vi "Send Subscription List To Robot.vi"(8 "error in (no error)":errorcluster, 10 "Selected parameters 2":refnum<vi>) -> (0 "error out":errorcluster)   [LabVIEW 2016]
uses:
  Communication Global variables.vi
  <vilib>/addons/_JKI.lib/REST Client/classes/REST Client/REST Client.lvclass
  <vilib>/addons/_JKI.lib/Serialization/JSON/JKI JSON Serialization.lvlib
panel:
  in  "Subscription list":T1={"type"="start", "subscription"=[]}
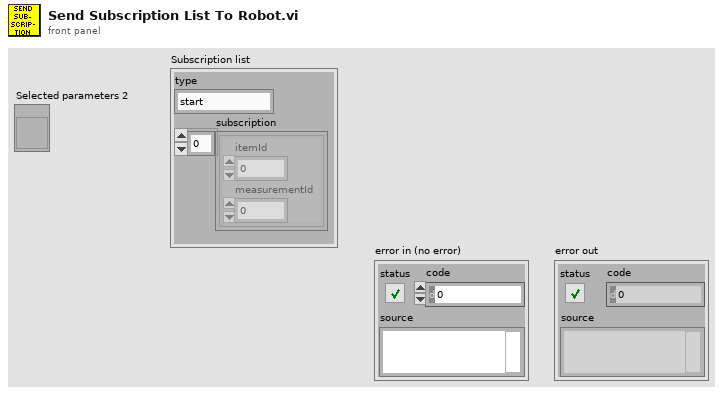
[diagram p1: front panel]
types:
  T1 = cluster{"type":string, "subscription":cluster{"itemId":i32, "measurementId":i32}[]}
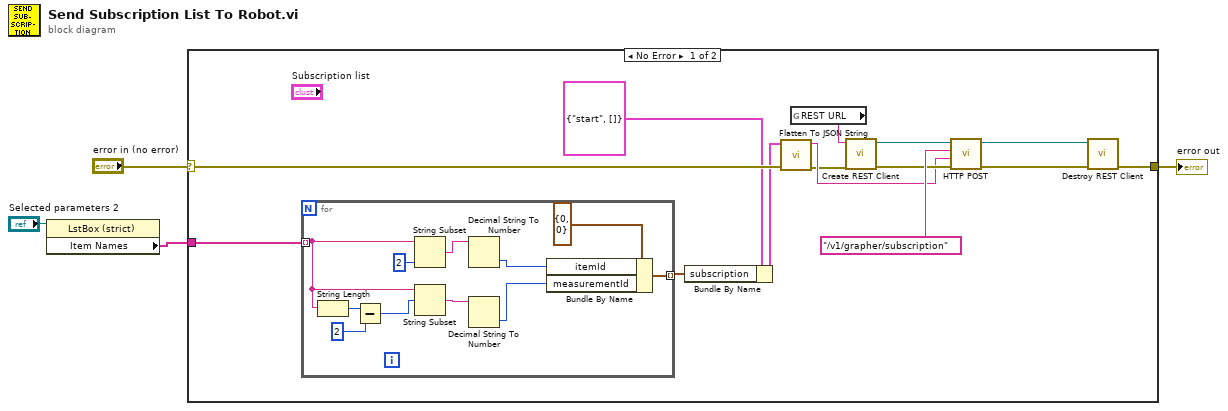
[diagram p0: block diagram]
diagram:
  n1 = property class="LstBox (strict)"(reference="Selected parameters 2") -> ("Item Names"=w1:string[])  [unwired: 1 in, 2 out]
  n2 = case shown="No Error" "error in (no error)" {
    selector: "error in (no error)" -> [w10 w30]
    tunnel: [w11 w30] -> w3
    tunnel: w1 -> [w5 _]
    frame No Error {
      n3 = for {
        tunnel: w5 -> [w25] mode=indexing
        tunnel: [w19] -> w7 mode=indexing
        n4 = String Length(string=w25) -> (length=w24:i32)
        n5 = Subtract(x=w24, y=2) -> (x-y=w22:i32)
        n6 = String Subset(string=w25, length (rest)=2 ("length (rest)")) -> (substring=w27:string)  [unwired: 1 in]
        n7 = String Subset(string=w25, offset (0)=w22) -> (substring=w21:string)  [unwired: 1 in]
        n8 = Decimal String To Number(string=w27) -> (number=w26:i32)  [unwired: 2 in, 1 out]
        n9 = Decimal String To Number(string=w21) -> (number=w20:i32)  [unwired: 2 in, 1 out]
        n10 = Bundle By Name(cluster=cluster{"itemId":i32, "measurementId":i32} {"itemId"=0, "measurementId"=0}, "itemId"=w26, "measurementId"=w20) -> (w19:cluster{"itemId":i32, "measurementId":i32})
      }
      n11 = Bundle By Name(cluster=T1 {"type"="start", "subscription"=[]} ("Subscription list"), "subscription"=w7) -> (w6:T1)
      n12 = call <vilib>:"Flatten To JSON String.vi"("error in (no error)"=w10, "Variant"=w6) -> ("error out"=w9:errorcluster, "JSON String"=w13:string)  [unwired: 8 in]
      n13 = global read "Communication Global variables.vi" "REST URL"() -> (w14:string)
      n14 = call <vilib>:"Create REST Client.vi"("error in (no error)"=w9, "Base URL"=w14) -> ("error out"=w16:errorcluster, "REST Client out"=w18:refnum<class "REST Client.lvclass">)  [unwired: 8 in]
      n15 = call-dynamic "HTTP POST.vi"("error in (no error)"=w16, "Request body"=w13, "Path"="/v1/grapher/subscription", "REST Client in"=w18) -> ("error out"=w12:errorcluster, "REST Client out"=w15:refnum<class "REST Client.lvclass">)  [unwired: 2 in, 4 out]
      n16 = call-dynamic "Destroy REST Client.vi"("error in (no error)"=w12, "REST Client in"=w15) -> ("error out"=w11:errorcluster)  [unwired: 9 in]
    }
    frame Error {
    }
  }
  "error out" <- w3
